vi "Controller_3_2_Proportional.vi"() -> ()   [LabVIEW 2019]
uses:
  <vilib>/myRIO/Instrument Drivers/Onboard IO/PWM/typedefs/PWM Configuration.ctl
  <vilib>/myRIO/Instrument Drivers/Onboard IO/PWM/PWM.lvlib
  <vilib>/myRIO/Common/Instrument Driver Framework/myRIO v1.0/PWM/typedefs/PWM Channels Enum.ctl
  <vilib>/myRIO/Common/Instrument Driver Framework/Utilities/typedefs/Generic FPGA Reference.ctl
  <vilib>/myRIO/Common/Instrument Driver Framework/Utilities/typedefs/myRIO v1.0 Reference.ctl
  <vilib>/myRIO/Common/Instrument Driver Framework/Utilities/typedefs/Hardware Version Enum.ctl
  <vilib>/myRIO/Common/Instrument Driver Framework/Utilities/typedefs/myRIO Generic Hardware Reference.ctl
  <vilib>/myRIO/Instrument Drivers/Onboard IO/PWM/typedefs/PWM Reference.ctl
  <vilib>/myRIO/Instrument Drivers/Onboard IO/PWM/vis/Set Duty Cycle and Frequency.vi
  <vilib>/userDefined/High Color/nirio_resource_hc.ctl
  <vilib>/myRIO/Common/Instrument Driver Framework/myRIO v1.0/PWM/vis/myRIO v1.1 Open PWM.vi
  <vilib>/myRIO/Instrument Drivers/Onboard IO/PWM/vis/myRIO PWM Open.xnode
  <vilib>/myRIO/Common/Instrument Driver Framework/Utilities/vis/Is FPGA Ref Available.vi
  <vilib>/myRIO/Express VI/Onboard IO/PWM/PWM Express VI.xnode
  <vilib>/myRIO/Common/Instrument Driver Framework/Utilities/typedefs/Analog Scaling Constants.ctl
  <vilib>/myRIO/Common/Instrument Driver Framework/Utilities/typedefs/Analog Scaling Constants List.ctl
  <vilib>/myRIO/Common/Instrument Driver Framework/myRIO v1.0/AI/typedefs/AI Channels Enum.ctl
  <vilib>/myRIO/Common/Instrument Driver Framework/myRIO v1.0/AI/typedefs/AI Channels List.ctl
  <vilib>/myRIO/Instrument Drivers/Onboard IO/AI/typedefs/AI Reference.ctl
  <vilib>/myRIO/Instrument Drivers/Onboard IO/AI/AI.lvlib
  <vilib>/myRIO/Instrument Drivers/Onboard IO/AI/vis/Read.vi
  <vilib>/myRIO/Common/Instrument Driver Framework/myRIO v1.0/AI/vis/myRIO v1.1 Open AI.vi
  <vilib>/myRIO/Instrument Drivers/Onboard IO/AI/vis/myRIO AI Open.xnode
  <vilib>/myRIO/Express VI/Onboard IO/AI/AI Express VI.xnode
  <vilib>/imath/engines/lvmath2/RunTimeEngine/Managers/WorkSpace/UID Generator.vi
  <vilib>/imath/engines/lvmath2/RunTimeEngine/LocalVariableDefStatement/MC_LocalVariableDefStatement_Display.vi
  <vilib>/imath/engines/lvmath2/RunTimeEngine/RunTimeType/NIMS_RunTimeType_From StrictType (excl LVString).vi
  <vilib>/imath/engines/lvmath2/RunTimeEngine/Managers/SymbolTable/Clear UID.vi
  <vilib>/imath/engines/lvmath2/RunTimeEngine/Managers/SymbolTable/NIMS_WorkSpace.lvlib
  <vilib>/imath/engines/lvmath2/RunTimeEngine/NodeEndStatement/NIMS_NodeEndStatement_Output.vi
  <vilib>/imath/engines/lvmath2/RunTimeEngine/ErrorHandling/NIMS_Finalize Error.vi
  <vilib>/addons/control/pid/NI_PID_pid.lvlib
  <vilib>/ptbypt/NI_PtbyPt.lvlib
  <vilib>/myRIO/Instrument Drivers/Utilities/Utilities.lvlib
  <vilib>/myRIO/Common/Instrument Driver Framework/myRIO v1.0/DIO/typedefs/DIO Channels Enum.ctl
  <vilib>/myRIO/Common/Instrument Driver Framework/myRIO v1.0/DIO/typedefs/DIO Channels List.ctl
  <vilib>/myRIO/Instrument Drivers/Onboard IO/DIO/typedefs/DIO Reference.ctl
  <vilib>/myRIO/Instrument Drivers/Onboard IO/DIO/DIO.lvlib
  <vilib>/myRIO/Instrument Drivers/Onboard IO/DIO/vis/Write.vi
  <vilib>/myRIO/Common/Instrument Driver Framework/myRIO v1.0/DIO/vis/myRIO v1.1 Open DIO.vi
  <vilib>/myRIO/Instrument Drivers/Onboard IO/DIO/vis/myRIO DIO Open.xnode
  <vilib>/myRIO/Express VI/Onboard IO/DO/DO Express VI.xnode
  <vilib>/addons/control/pid/pid.llb/PID (DBL).vi
  <vilib>/Simulation/Implementation/XNodeFramework/SimXNode/SimX.xnode
  Subsystems/Graph_2_Signal.vi
  <vilib>/Simulation/Implementation/Shared/SIMSCR Execution Mode.ctl
  <vilib>/Simulation/Scripting/Companion Diagram/SimConfigNode/_simSolvers.ctl
  <vilib>/Simulation/Scripting/Companion Diagram/SimConfigNode/SimParams.ctl
  <vilib>/Simulation/Scripting/Companion Diagram/SimConfigNode/SimDog.xnode
  Subsystems/Graph_3_Signal.vi
  <vilib>/Simulation/Implementation/Shared/SIM Bundle Sim Info.vi
  <vilib>/Simulation/Implementation/Shared/SIM Unbundle Sim Info.vi
  <vilib>/Simulation/Implementation/Shared/NILVSim_FinalizeModel.vi
  <vilib>/Simulation/Implementation/Shared/NILVSim_GetModelError.vi
  <vilib>/Simulation/Implementation/Shared/NILVSim_Initialize.vi
  <vilib>/Simulation/Utility/Implementation/NILVSim Get Time and IsAcceptedStep.vi
  <vilib>/Simulation/Implementation/Shared/NILVSim_Manager.vi
  <vilib>/Simulation/Implementation/Shared/NI_SIM_Implementation.lvlib
  <vilib>/Simulation/Implementation/Shared/NILVSIM_BeginStep.vi
  <vilib>/Simulation/Param Hierarchy/Typedefs/SIMPH Param Control Actions.ctl
  <vilib>/Simulation/Implementation/Shared/NILVSim_ParamChanged.vi
  <vilib>/Utility/error.llb/Clear Errors.vi
  <vilib>/Simulation/Implementation/Shared/SIMSH Read Queue.vi
panel:
  out "Duty Cycle":dynamicdata(graph)
  out "Pressure Actuator":dynamicdata(graph)
  out "Pressure Motor":dynamicdata(graph)
  out "Pressures Actuator":cluster{dbl, dbl}(knob)={0.0, 8.870406975580165} scale=0.0..120.0
  in  "stop":bool
  out "VA_sensor":dbl format="%#.3g"
  out "Pressures Receiver":cluster{dbl, dbl}(knob)={0.0, 8.870406975580165} scale=0.0..120.0
  in  "Setpoint Preceiver":dbl(slide) scale=0.0..80.0
  out "V_Rsensor":dbl format="%#.3g"
  in  "PID Motor":T1={"proportional gain (Kc)"=0.01, "integral time (Ti, min)"=0.005, "derivative time (Td, min)"=0.0} {"derivative time (Td, min)" format="%.3f"; "integral time (Ti, min)" format="%.3f"; "proportional gain (Kc)" format="%.3f"}
  out "Duty cycle Motor":dbl(knob) scale=0.0..1.0
  in  "Setpoint Pactuator":dbl(slide) scale=0.0..70.0
  in  "milliseconds to wait":u32=100
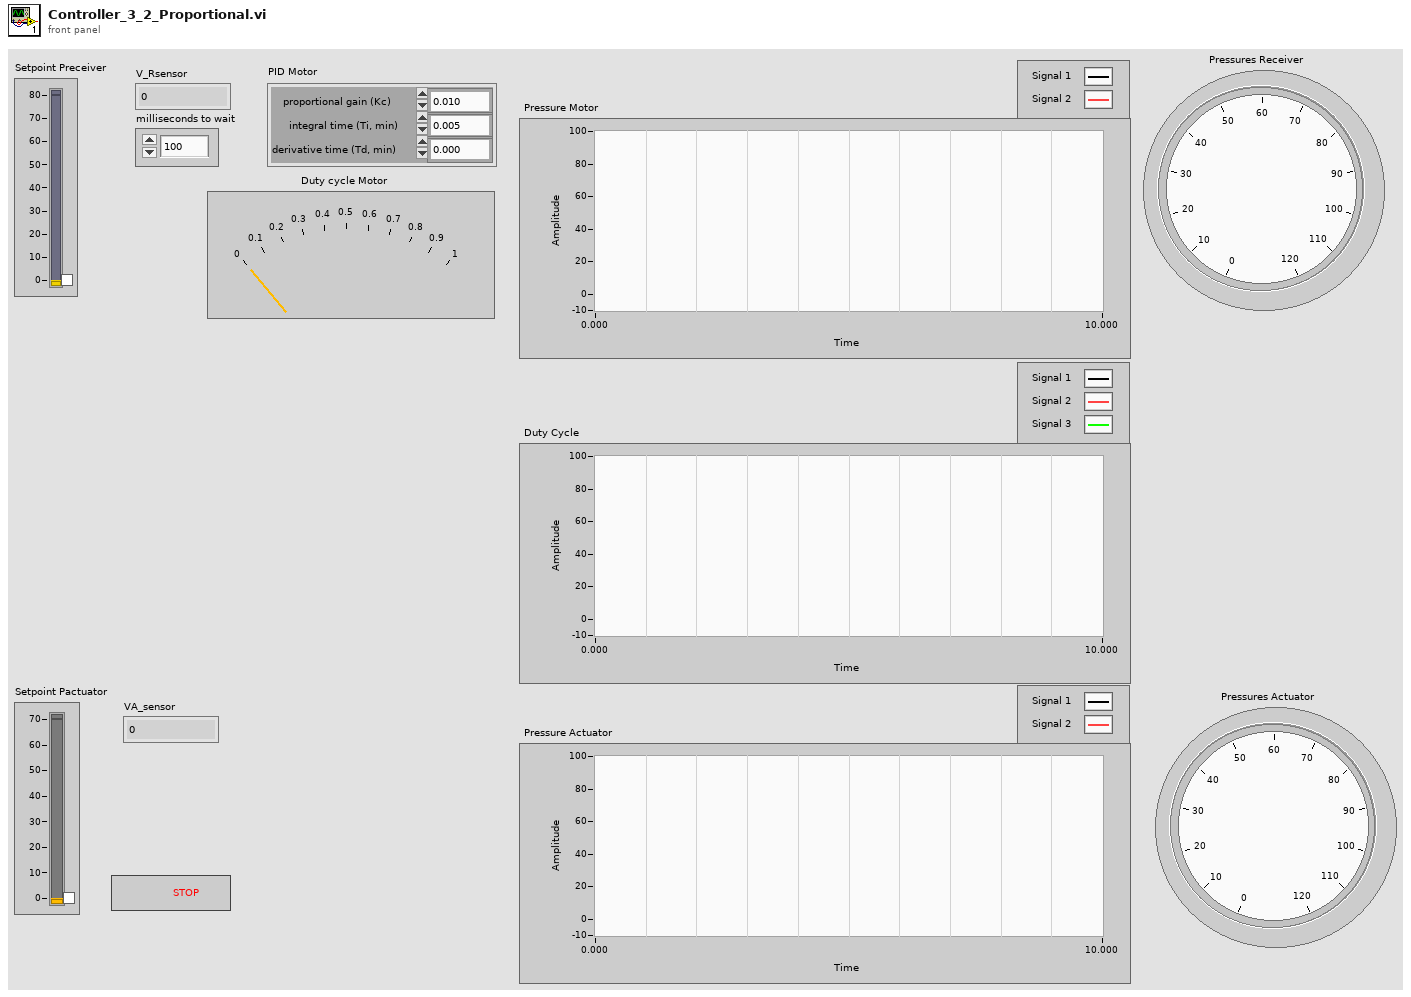
[diagram p1: front panel]
types:
  T1 = cluster{"proportional gain (Kc)":dbl, "integral time (Ti, min)":dbl, "derivative time (Td, min)":dbl}
  T2 = enum16{"Simulate to Completion", "Single Time-Step Simulation (Fixed Step Only)"}
  T3 = typedef "SIMSCR Execution Mode.ctl" = enum16{"Simulate to Completion", "Single Time-Step Simulation (Fixed Step Only)"}
  T4 = typedef "SIMPH Param Control Actions.ctl" = enum16{"get params", "set params"}
  T5 = typedef "SimParams.ctl" = cluster{"Initial Time (s)":dbl, "Final Time (s)":dbl, "Step Size (s)":dbl, "ODE Solver":T6, "Minimum Step Size (s)":dbl, "Maximum Step Size (s)":dbl, "Relative Tolerance":dbl, "Absolute Tolerance":dbl, "Software Timing":bool, "Initial Step Size (s)":dbl, "Automatic Fixed Step Size?":bool, "Automatic Discrete Step Size?":bool, "Discrete Step Size (s)":dbl, "Calculate using Time Step":bool, "Solver Wired?":bool, "Prev.Frm.Expected End":u64, "Prev.Frm.Actual End":u64, "Prev.Frm.Finished Late?":bool, "Prev.Iter.Expected End":u64, "Prev.Iter.Actual End":u64, "Prev.Iter.Finished Late?":bool, "Expected Iteration Start":u64, "Actual Iteration Start":u64, "Expected Frame Start":u64, "Actual Frame Start":u64, "Source Name":string, "Name":string, "Period":i64, "Deadline":i64, "Offset":i64, "Start":i64, "Priority":i32, "Timeout":i32, "Processor":i32, "Mode":enum32{"No Change", "Process missed periods, maintain original phase", "Discard missed periods, maintain original phase", "Process missed periods, ignore original phase", "Discard missed periods, ignore original phase"}, "Wakeup reason":enum32{"Normal", "Aborted", "Asynchronous wakeup", "Timing source error", "Timed loop error", "Timeout"}, "Error":errorcluster, "Source Type":string, "Secondary Source Type":string, "Global End Time":u64, "Global Start Time":u64, "Full Solver Reset":bool, "Execution Mode":T3, "Nan/Inf Check":bool, "Custom Solver Library":string, "Solver Is Variable":bool, "custom solver name":string, "Signal Collection Decimation":u32}
  T6 = typedef "_simSolvers.ctl" = enum16{"Runge-Kutta 1 (Euler)", "Runge-Kutta 2", "Runge-Kutta 3", "Runge-Kutta 4", "Runge-Kutta 23 (variable)", "Runge-Kutta 45 (variable)", "BDF (variable)", "Adams-Moulton (variable)", "Rosenbrock (variable)", "Discrete States Only", "SDIRK 4 (variable)", "Radau 5 (variable)", "Radau 9 (variable)", "Radau 13 (variable)", "Radau [Variable Order] (variable)", "Gear's Method (variable)", "Linearizer", "State Query", "Trim Eval", "Custom Solver"}
  T7 = typedef "DIO.lvlib/DIO Reference.ctl" = cluster{"myRIO Reference":T8, "DIO Channels List":T12}
  T8 = typedef "myRIO Generic Hardware Reference.ctl" = cluster{"myRIO Model":T9, "myRIO Hardware Reference":T10}
  T9 = typedef "Hardware Version Enum.ctl" = enum16{"Unknown", "myRIO-1900", "myRIO-1950", "roboRIO", "NI ELVIS RIO CM", "ELVIS III"}
  T10 = typedef "myRIO v1.0 Reference.ctl" = cluster{"Generic FPGA Reference":T11, "Allow multiple opens":bool}
  T11 = typedef "Generic FPGA Reference.ctl" = refnum<k20>
  T12 = typedef "DIO Channels List.ctl" = T13[]
  T13 = typedef "DIO Channels Enum.ctl" = enum16{"Not Connected", "C/DIO0", "C/DIO1", "C/DIO2", "C/DIO3", "C/DIO4", "C/DIO5", "C/DIO6", "C/DIO7", "A/DIO0", "A/DIO1", "A/DIO2", "A/DIO3", "A/DIO4", "A/DIO5", "A/DIO6", "A/DIO7", "A/DIO8", "A/DIO9", "A/DIO10", "A/DIO11", "A/DIO12", "A/DIO13", "A/DIO14", "A/DIO15", "A/DIO16", "A/DIO17", "A/DIO18", "A/DIO19", "B/DIO0", "B/DIO1", "B/DIO2", "B/DIO3", "B/DIO4", "B/DIO5", "B/DIO6", "B/DIO7", "B/DIO8", "B/DIO9", "B/DIO10", "B/DIO11", "B/DIO12", "B/DIO13", "B/DIO14", "B/DIO15", "B/DIO16", "B/DIO17", "B/DIO18", "B/DIO19", "LED0", "LED1", "LED2", "LED3", "Button0", "DIO/DIO0", "DIO/DIO1", "DIO/DIO2", "DIO/DIO3", "DIO/DIO4", "DIO/DIO5", "DIO/DIO6", "DIO/DIO7", "DIO/DIO8", "DIO/DIO9", "SPI/CS0", "SPI/CS1", "SPI/CS2", "SPI/CS3", "LED RADIO (Green)", "LED RADIO (Red)", "LED COMM (Green)", "LED COMM (Red)", "LED MODE (Green)", "LED MODE (Red)"}
  T14 = typedef "nirio_resource_hc.ctl" = tag
  T15 = typedef "AI.lvlib/AI Reference.ctl" = cluster{"myRIO Reference":T8, "AI Channels List":T16, "AI Scaling Constants List":T18}
  T16 = typedef "AI Channels List.ctl" = T17[]
  T17 = typedef "AI Channels Enum.ctl" = enum16{"Not Connected", "AudioIn/Left", "AudioIn/Right", "C/AI0", "C/AI1", "A/AI0", "A/AI1", "A/AI2", "A/AI3", "A/AI4", "A/AI5", "A/AI6", "A/AI7", "B/AI0", "B/AI1", "B/AI2", "B/AI3", "B/AI4", "B/AI5", "B/AI6", "B/AI7", "AI/AI0", "AI/AI1", "AI/AI2", "AI/AI3", "A/AI0 (DIFF)", "A/AI1 (DIFF)", "A/AI2 (DIFF)", "A/AI3 (DIFF)", "B/AI0 (DIFF)", "B/AI1 (DIFF)", "B/AI2 (DIFF)", "B/AI3 (DIFF)"}
  T18 = typedef "Analog Scaling Constants List.ctl" = T19[]
  T19 = typedef "Analog Scaling Constants.ctl" = cluster{"LSB Weight (Volts)":dbl, "Offset (Volts)":dbl, "Signed?":bool}
  T20 = typedef "PWM.lvlib/PWM Reference.ctl" = cluster{"myRIO Reference":T8, "PWM Channels Enum":T21, "PWM Configuration":T22}
  T21 = typedef "PWM Channels Enum.ctl" = enum16{"Not Connected", "C/PWM0", "C/PWM1", "A/PWM0", "A/PWM1", "A/PWM2", "A/PWM3", "A/PWM4", "A/PWM5", "A/PWM6", "A/PWM7", "A/PWM8", "A/PWM9", "A/PWM10", "A/PWM11", "A/PWM12", "A/PWM13", "A/PWM14", "A/PWM15", "A/PWM16", "A/PWM17", "A/PWM18", "A/PWM19", "B/PWM0", "B/PWM1", "B/PWM2", "B/PWM3", "B/PWM4", "B/PWM5", "B/PWM6", "B/PWM7", "B/PWM8", "B/PWM9", "B/PWM10", "B/PWM11", "B/PWM12", "B/PWM13", "B/PWM14", "B/PWM15", "B/PWM16", "B/PWM17", "B/PWM18", "B/PWM19", "PWM/PWM0", "PWM/PWM1", "PWM/PWM2", "PWM/PWM3", "PWM/PWM4", "PWM/PWM5", "PWM/PWM6", "PWM/PWM7", "PWM/PWM8", "PWM/PWM9"}
  T22 = typedef "PWM.lvlib/PWM Configuration.ctl" = cluster{"Frequency":dbl, "Duty Cycle":dbl}
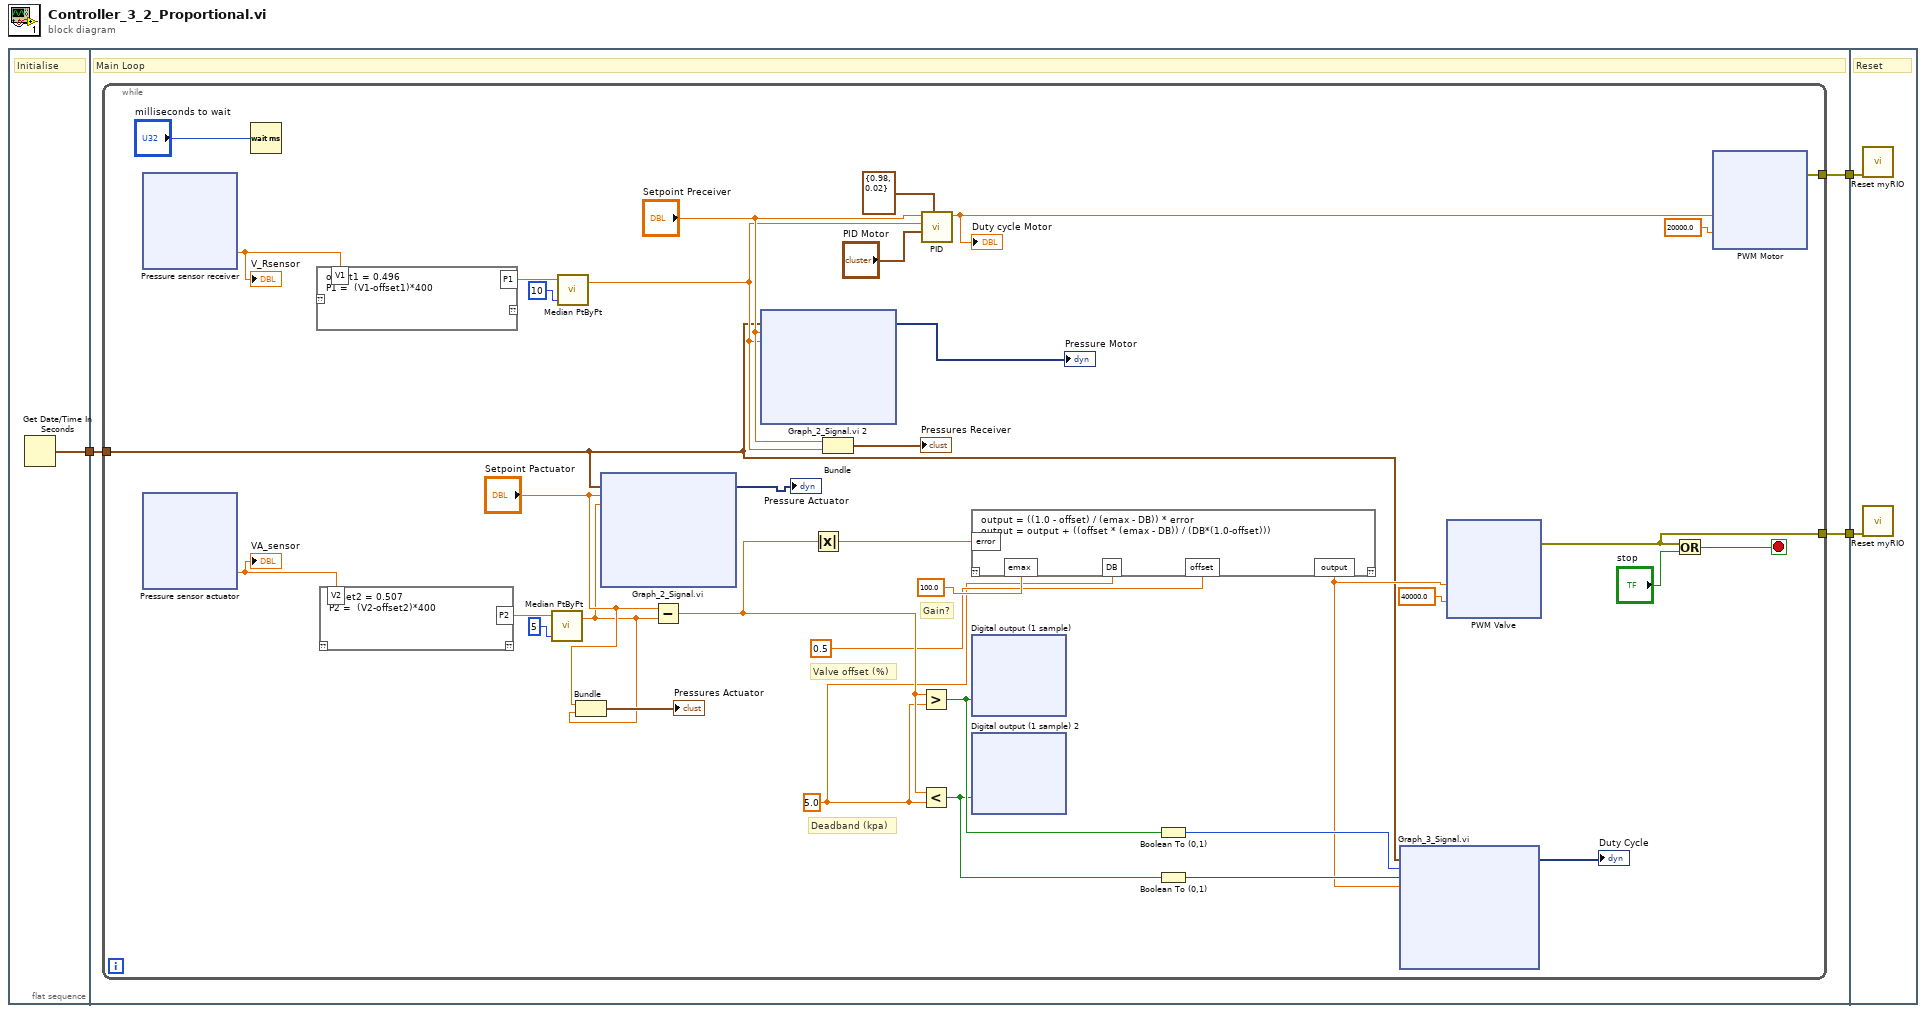
[diagram p0: block diagram]
diagram:
  n1 = flat-sequence {
    tunnel: [w4] -> w3
    tunnel: [w7] -> w2
    tunnel: [w6] -> w1
    tunnel: w3 -> [w5]
    tunnel: w2 -> [w1190]
    tunnel: w1 -> [w1189]
    frame #0 {
      # "Initialise"
      n2 = Get Date/Time In Seconds() -> (seconds since 1Jan1904=w4:timestamp)
    }
    frame #1 {
      # "Main Loop"
      n3 = while {
        tunnel: [w42] -> w7
        tunnel: [w31] -> w6
        tunnel: w5 -> [w14]
        stop <- w41 stop-if-true
        w22 = 5.0 ("Frequency [Hz]")
        # "Valve offset (%)"
        # "Deadband (kpa)"
        # "Gain?"
        n4 = xnode "Pressure sensor receiver"() -> ("A/AI1 (Pin 5)"=w30:dbl)  [unwired: 1 in, 1 out]
        "V_Rsensor" <- w30
        n5 = xnode "Pressure sensor actuator"() -> ("A/AI0 (Pin 3)"=w40:dbl)  [unwired: 1 in, 1 out]
        "VA_sensor" <- w40
        n6 = Wait (ms)(milliseconds to wait="milliseconds to wait") -> ()  [unwired: 1 out]
        n7 = mathscript code="offset1 = 0.496\nP1 =  (V1-offset1)*400"("V1"=w30) -> ("P1"=w33:dbl)  [unwired: 1 in, 1 out]
        n8 = mathscript code="offset2 = 0.507\nP2 =  (V2-offset2)*400"("V2"=w40) -> ("P2"=w39:dbl)  [unwired: 1 in, 1 out]
        n9 = call <vilib>:"Median PtByPt.vi"("sample length"=5, "x"=w39) -> ("median"=w11:dbl)  [unwired: 2 in, 1 out]
        n10 = call <vilib>:"Median PtByPt.vi"("sample length"=10, "x"=w33) -> ("median"=w15:dbl)  [unwired: 2 in, 1 out]
        n11 = Bundle("Setpoint Pactuator"="Setpoint Pactuator", "median"=w11) -> (→"Pressures Actuator":cluster{"Setpoint Pactuator":dbl, "median":dbl})  [unwired: 1 in]
        n12 = xnode "Graph_2_Signal.vi"("y"=w14, "Dynamic Data 2"="Setpoint Pactuator", "Dynamic Data 1"=w11) -> ("Signals"=→"Pressure Actuator":dynamicdata)  [unwired: 2 in, 9 out]
        n13 = Subtract(x="Setpoint Pactuator", y=w11) -> (x-y=w26:dbl)
        n14 = xnode "Graph_2_Signal.vi 2"("y"=w14, "Dynamic Data 2"="Setpoint Preceiver", "Dynamic Data 1"=w15) -> ("Signals"=→"Pressure Motor":dynamicdata)  [unwired: 2 in, 9 out]
        n15 = Absolute Value(x=w26) -> (abs(x)=w25:dbl)
        n16 = Bundle("Setpoint Preceiver"="Setpoint Preceiver", "median"=w15) -> (→"Pressures Receiver":cluster{"Setpoint Preceiver":dbl, "median":dbl})  [unwired: 1 in]
        n17 = Greater?(x=w26, y=w22) -> (0:w21:bool)
        n18 = Less?(x=w26, y=w22) -> (x < y?=w20:bool)
        n19 = call-poly <vilib>:"PID.vi"("output range"=cluster{"output high":dbl, "output low":dbl} {"output high"=0.98, "output low"=0.02} ("output range motor"), "PID gains"="PID Motor", "process variable"=w15, "setpoint"="Setpoint Preceiver") -> ("output"=w29:dbl)  [unwired: 6 in, 1 out]
        "Duty cycle Motor" <- w29
        n20 = mathscript code="output = ((1.0 - offset) / (emax - DB)) * error\noutput = output + ((offset * (emax - DB)) / (DB*(1.0-offset)))"("error"=w25, "offset"=0.5 ("Frequency [Hz]"), "emax"=100.0 ("Frequency [Hz]"), "DB"=w22) -> ("output"=w17:dbl)  [unwired: 1 in, 1 out]
        n21 = xnode "Digital output (1 sample)"("B/DIO0 (Pin 11)"=w21) -> ()  [unwired: 1 in, 1 out]
        n22 = xnode "Digital output (1 sample) 2"("B/DIO0 (Pin 11)"=w20) -> ()  [unwired: 1 in, 1 out]
        n23 = Boolean To (0,1)(Boolean=w21) -> (0, 1=w19:i16)
        n24 = Boolean To (0,1)(Boolean=w20) -> (0, 1=w18:i16)
        n25 = xnode "Graph_3_Signal.vi"("y"=w14, "Dynamic Data 3"=w19, "Dynamic Data Type 2"=w18, "Dynamic Data Type"=w17) -> ("Signals"=→"Duty Cycle":dynamicdata)  [unwired: 2 in, 8 out]
        n26 = xnode "PWM Valve"("Duty Cycle"=w17, "Frequency [Hz]"=40000.0) -> ("error out"=w42:errorcluster)  [unwired: 1 in]
        n27 = Or(x=w42, y="stop") -> (x .or. y?=w41:bool)
        n28 = xnode "PWM Motor"("Duty Cycle"=w29, "Frequency [Hz]"=20000.0) -> ("error out"=w31:errorcluster)  [unwired: 1 in]
      }
    }
    frame #2 {
      # "Reset"
      n29 = call <vilib>:"Reset myRIO.vi"("error in (no error)"=w1189) -> ()  [unwired: 10 in, 1 out]
      n30 = call <vilib>:"Reset myRIO.vi"("error in (no error)"=w1190) -> ()  [unwired: 10 in, 1 out]
    }
  }
